vi "labview_analog_voltage_io_example.vi"() -> ()   [LabVIEW 2017]
uses:
  <vilib>/DAQmx/write.llb/DAQmx Write (Analog DBL 1Chan 1Samp).vi
  <vilib>/DAQmx/read.llb/DAQmx Read (Analog DBL 1Chan 1Samp).vi
  <vilib>/DAQmx/miscellaneous.llb/DAQmx Fill In Error Info.vi
panel:
  out "AI [V]":dbl(knob) scale=0.0..5.0
  in  "AO [V]":dbl(slide) scale=0.0..5.0
  in  "Stop Button":bool
  # "Analog voltage I/O with NI USB-6008 Example"
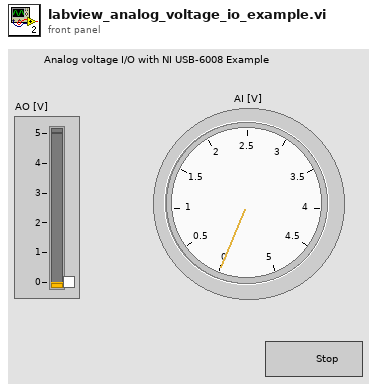
[diagram p1: front panel]
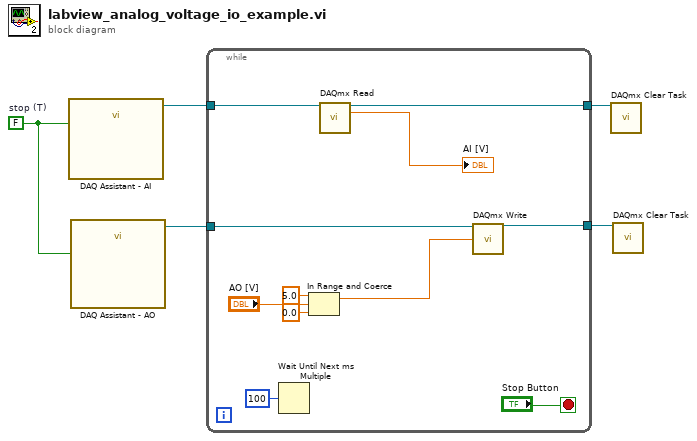
[diagram p0: block diagram]
diagram:
  w5 = FALSE  # stop (T)
  n1 = call "DAQ Assistant - AI"("stop (T)"=w5) -> ("task out"=w3:refnum<k21>)  [unwired: 3 in, 15 out]
  n2 = call "DAQ Assistant - AO"("stop (T)"=w5) -> ("task out"=w4:refnum<k21>)  [unwired: 4 in, 14 out]
  n3 = while {
    tunnel: w3 -> [w16]
    tunnel: w4 -> [w13]
    tunnel: [w10] -> w2
    tunnel: [w9] -> w1
    stop <- "Stop Button" stop-if-true
    n4 = Wait Until Next ms Multiple(millisecond multiple=u32 100) -> ()  [unwired: 1 out]
    n5 = In Range and Coerce(upper limit=5.0, x="AO [V]", lower limit=0.0) -> (coerced(x)=w12:dbl)  [unwired: 1 out]
    n6 = call-poly <vilib>:"DAQmx Read.vi"("task/channels in"=w16) -> ("task out"=w10:refnum<k21>, "data"=→"AI [V]":dbl)  [unwired: 1 in, 12 out]
    n7 = call-poly <vilib>:"DAQmx Write.vi"("task/channels in"=w13, "data"=w12) -> ("task out"=w9:refnum<k21>)  [unwired: 2 in, 11 out]
  }
  n8 = call <vilib>:"DAQmx Clear Task.vi"("task in"=w2) -> ()  [unwired: 14 in, 1 out]
  n9 = call <vilib>:"DAQmx Clear Task.vi"("task in"=w1) -> ()  [unwired: 14 in, 1 out]
